vi "test no approved file exists fails.vi"(8 "error in":errorcluster, 11 "TestCase in":refnum<class "Testing Approval Tests.lvclass">) -> (0 "error out":errorcluster, 3 "TestCase out":refnum<class "Testing Approval Tests.lvclass">)   [LabVIEW 2020, in "Testing Approval Tests.lvclass"]
uses:
  Testing Approval Tests.lvclass
  <vilib>/addons/_JKI Toolkits/VI Tester/TestCase.llb/TestCase.lvclass
  Approval Tests/Approval Tests.lvlib
  C:/Program Files/National Instruments/LabVIEW 2020/vi.lib/addons/_JKI Toolkits/VI Tester/TestCase.llb/TestCase.lvclass
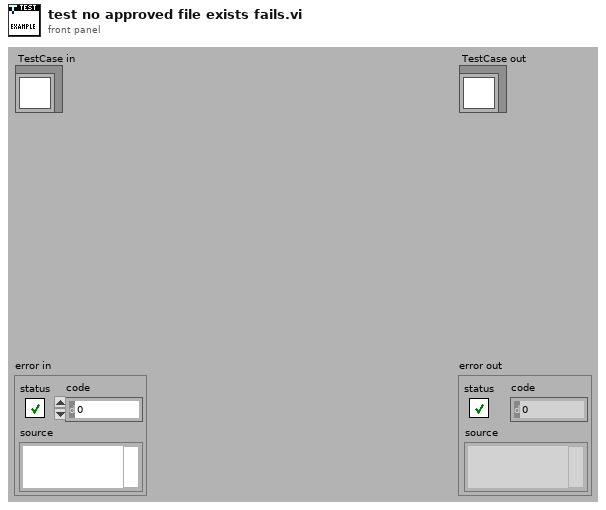
[diagram p1: front panel]
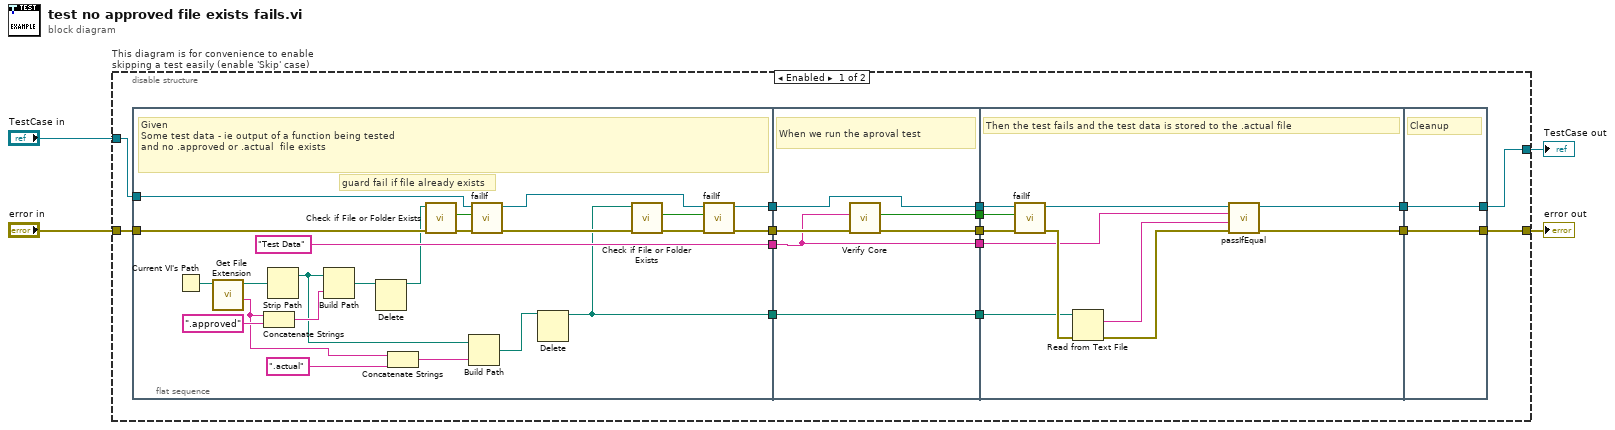
[diagram p0: block diagram]
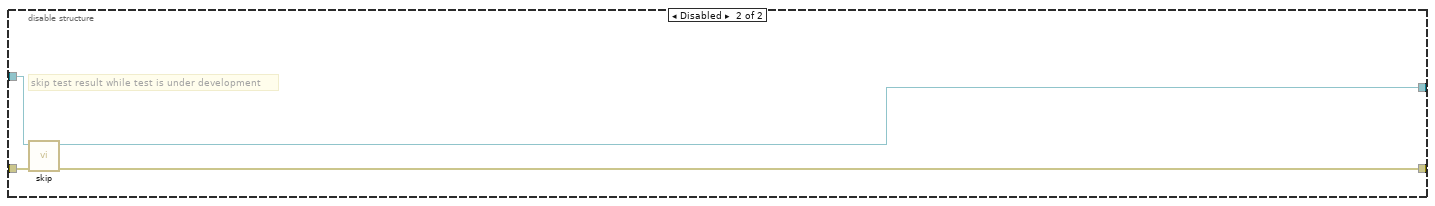
[diagram p2: hidden frame]
diagram:
  n1 = disable-structure "This diagram is for convenience to enable skipping a test easily (enable 'Skip' case)" shown="Enabled" {
    disable-tunnel: "TestCase in" -> [w12 w63]
    disable-tunnel: [w10 w62] -> w1
    disable-tunnel: [w16 w65] -> w3
    disable-tunnel: "error in" -> [w19 w64]
    frame Enabled {
      n2 = flat-sequence {
        tunnel: [w23] -> w13
        tunnel: w12 -> [w32]
        tunnel: w19 -> [w41]
        tunnel: [w39] -> w18
        tunnel: ["Test Data"] -> w8
        tunnel: [w21] -> w6
        tunnel: [w46] -> w14
        tunnel: w13 -> [w46]
        tunnel: w18 -> [w48]
        tunnel: [w47] -> w17
        tunnel: [w45] -> w9
        tunnel: w8 -> [w43]
        tunnel: [w44] -> w7
        tunnel: w6 -> [w44]
        tunnel: [w43] -> w5
        tunnel: w14 -> [w55]
        tunnel: [w51] -> w11
        tunnel: w17 -> [w59]
        tunnel: [w56] -> w15
        tunnel: w9 -> [w54]
        tunnel: w7 -> [w53]
        tunnel: w5 -> [w49]
        tunnel: w11 -> [w60]
        tunnel: [w60] -> w10
        tunnel: [w61] -> w16
        tunnel: w15 -> [w61]
        frame #0 {
          # "guard fail if file already exists"
          # "Given\nSome test data - ie output of a function being tested \nand no .approved or .actual  file exists"
          n3 = Current VI's Path() -> (path=w36:path)
          n4 = call <vilib>:"Get File Extension.vi"("file"=w36) -> ("filename without extension"=w20:string, "dup file"=w35:path)  [unwired: 6 in, 3 out]
          n5 = Concatenate Strings(w20, ".approved" ("string")) -> (w28:string)
          n6 = Strip Path(path=w35) -> (stripped path=w26:path)  [unwired: 1 out]
          n7 = Build Path(base path=w26, name or relative path=w28) -> (appended path=w33:path)
          n8 = Delete(path (use dialog)=w33) -> (deleted path=w31:path)  [unwired: 4 in, 2 out]
          n9 = Concatenate Strings(w20, ".actual" ("string")) -> (w27:string)
          n10 = call <vilib>:"Check if File or Folder Exists.vi"("error in (no error)"=w41, "path"=w31) -> ("error out"=w40:errorcluster, "file or folder exists?"=w30:bool)  [unwired: 7 in, 1 out]
          n11 = Build Path(base path=w26, name or relative path=w27) -> (appended path=w25:path)
          n12 = call-dynamic "failIf.vi"("error in (no error)"=w40, "fail"=w30, "TestCase in"=w32) -> ("error out"=w42:errorcluster, "TestCase out"=w24:refnum<class "Testing Approval Tests.lvclass">)  [unwired: 7 in]
          n13 = Delete(path (use dialog)=w25) -> (deleted path=w21:path)  [unwired: 4 in, 2 out]
          n14 = call <vilib>:"Check if File or Folder Exists.vi"("error in (no error)"=w42, "path"=w21) -> ("error out"=w38:errorcluster, "file or folder exists?"=w22:bool)  [unwired: 7 in, 1 out]
          n15 = call-dynamic "failIf.vi"("error in (no error)"=w38, "fail"=w22, "TestCase in"=w24) -> ("error out"=w39:errorcluster, "TestCase out"=w23:refnum<class "Testing Approval Tests.lvclass">)  [unwired: 7 in]
        }
        frame #1 {
          # "When we run the aproval test"
          n16 = call "Verify Core.vi"("error in"=w48, "Test Data"=w43) -> ("error out"=w47:errorcluster, "Passed?"=w45:bool)  [unwired: 7 in, 1 out]
        }
        frame #2 {
          # "Then the test fails and the test data is stored to the .actual file"
          n17 = call-dynamic "failIf.vi"("error in (no error)"=w59, "fail"=w54, "TestCase in"=w55) -> ("error out"=w58:errorcluster, "TestCase out"=w52:refnum<class "Testing Approval Tests.lvclass">)  [unwired: 7 in]
          n18 = Read from Text File(file (use dialog)=w53, error in=w58) -> (text=w50:string, error out=w57:errorcluster)  [unwired: 2 in, 2 out]
          n19 = call-dynamic "passIfEqual.vi"("error in (no error)"=w57, "y"=w50, "x"=w49, "TestCase in"=w52) -> ("error out"=w56:errorcluster, "TestCase out"=w51:refnum<class "Testing Approval Tests.lvclass">)  [unwired: 6 in]
        }
        frame #3 {
          # "Cleanup"
        }
      }
    }
    frame Disabled {
      # "skip test result while test is under development"
      n20 = call <vilib>:"skip.vi"("error in (no error)"=w64, "TestCase in"=w63) -> ("error out"=w65:errorcluster, "TestCase out"=w62:refnum<class "Testing Approval Tests.lvclass">)  [unwired: 8 in]
    }
  }
  "error out" <- w3
  "TestCase out" <- w1
